vi "data_read.vi"(9 "路径":path, 10 "感情数目":dbl, 11 "训练次数":dbl) -> (0 "字符串 2":string, 2 "输出簇":T2, 3 "字符串":string)   [LabVIEW 2014]
panel:
  out "错误输出 6":errorcluster caption="错误输出"
  out "错误输出 5":errorcluster caption="错误输出"
  out "字符串 6":string
  out "字符串 5":string
  out "输出簇 4":T1
  out "错误输出 4":errorcluster caption="错误输出"
  out "错误输出 3":errorcluster caption="错误输出"
  out "字符串 4":string
  out "字符串 3":string
  out "错误输出":errorcluster
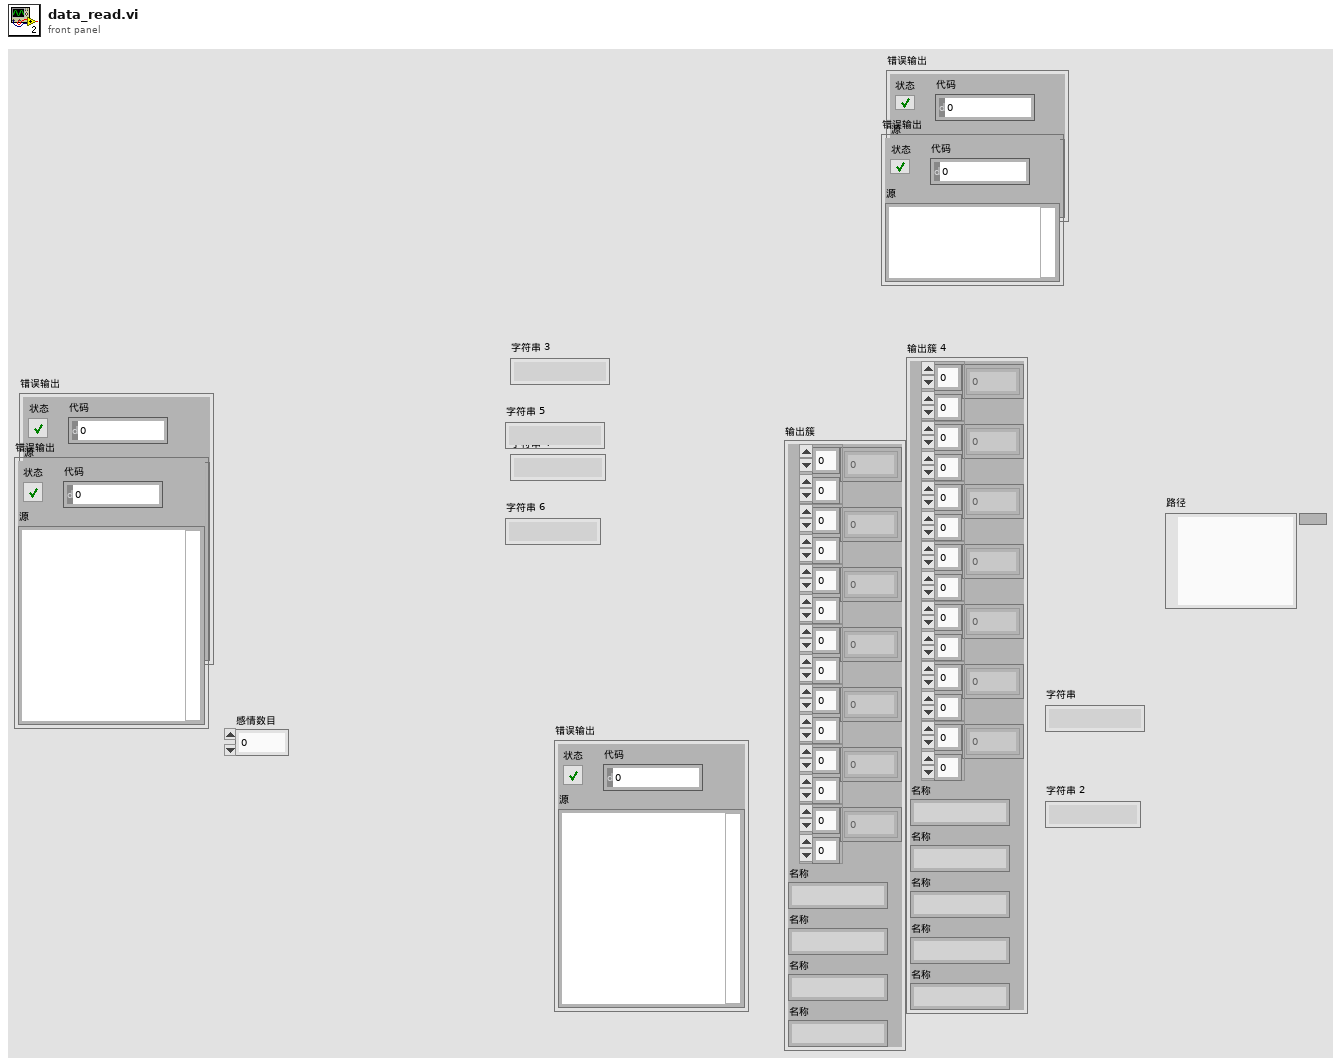
[diagram p1: front panel]
types:
  T1 = cluster{dbl[][], dbl[][], dbl[][], dbl[][], dbl[][], dbl[][], dbl[][], "名称":string, "名称":string, "名称":string, "名称":string, "名称":string}
  T2 = cluster{dbl[][], dbl[][], dbl[][], dbl[][], dbl[][], dbl[][], dbl[][], "名称":string, "名称":string, "名称":string, "名称":string}
  T3 = enum16{"open", "replace", "create", "open or create", "replace or create", "replace or create with confirmation"}
  T4 = cluster{dbl[][], dbl[][], dbl[][], dbl[][], dbl[][], dbl[][], dbl[][], "名称":string, "名称":string, "名称":string, "名称":string, "名称":string, "名称":string}
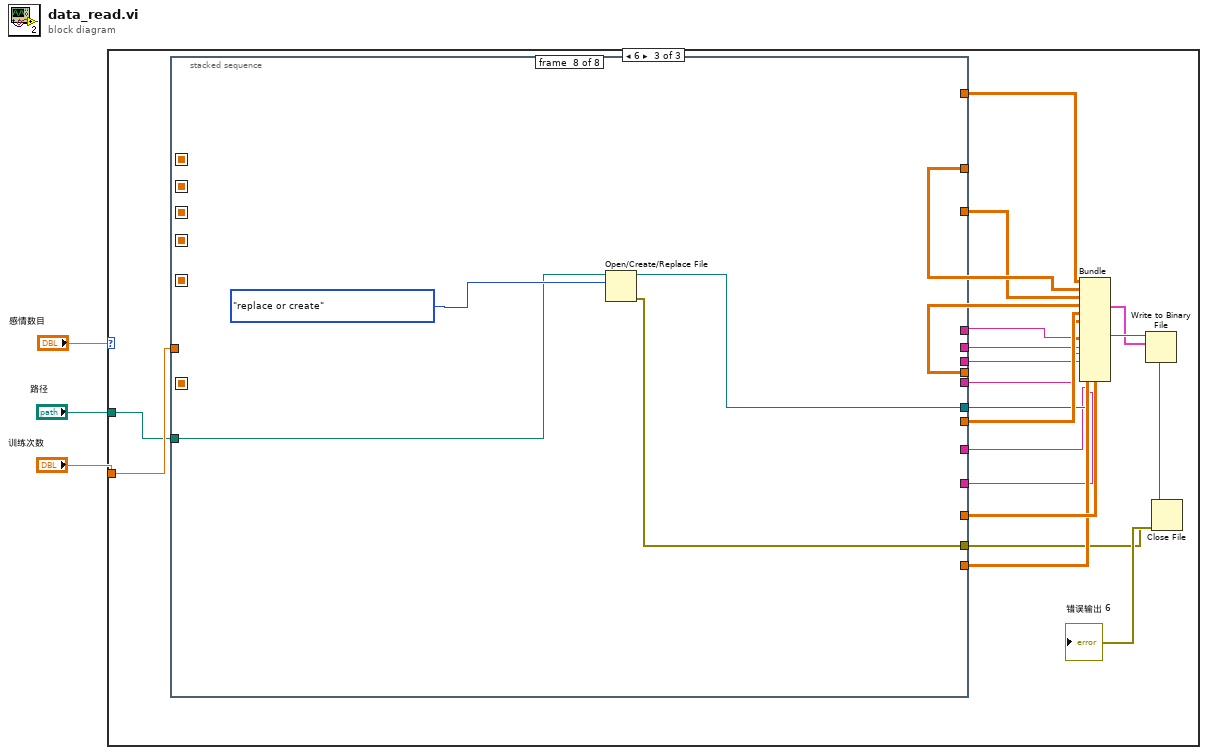
[diagram p0: block diagram]
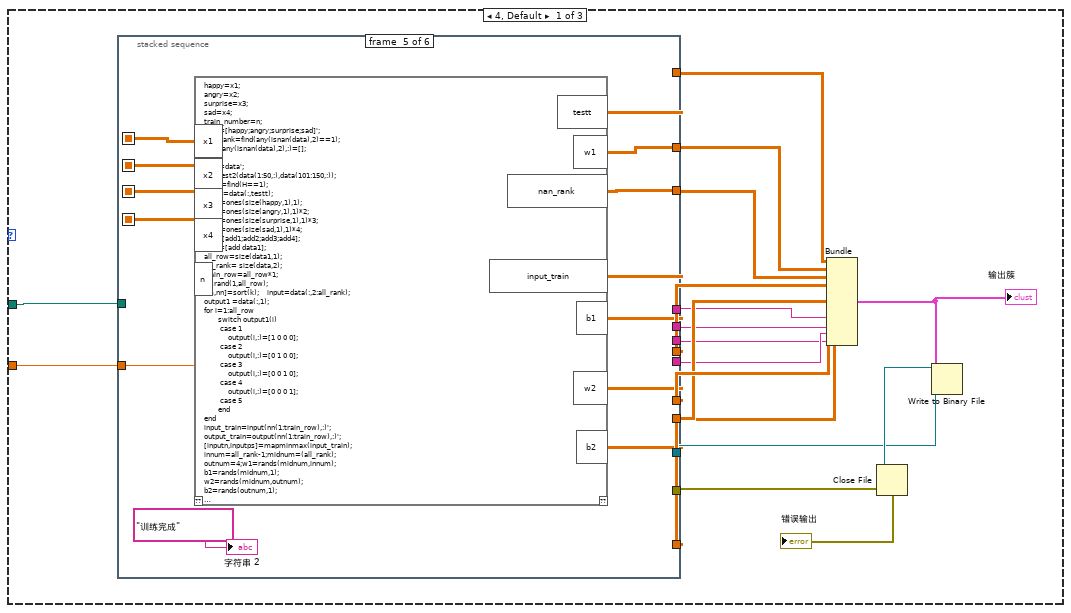
[diagram p2: hidden frame]
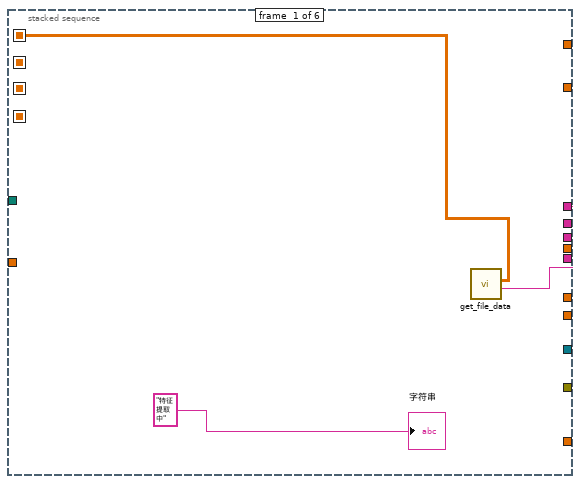
[diagram p3: hidden frame]
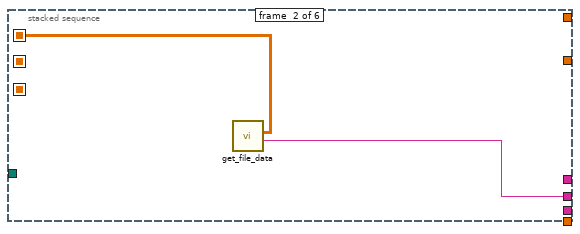
[diagram p4: hidden frame]
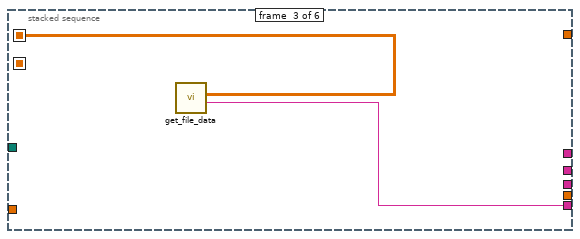
[diagram p5: hidden frame]
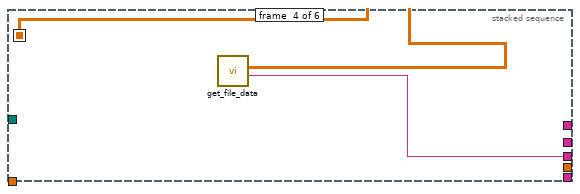
[diagram p6: hidden frame]
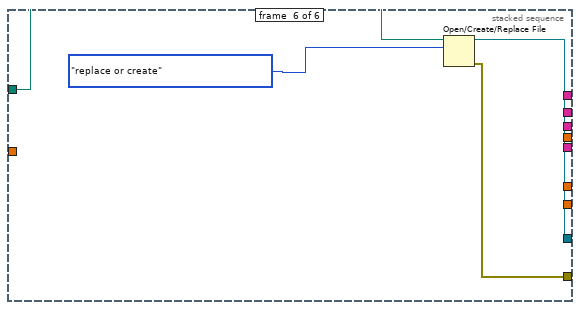
[diagram p7: hidden frame]
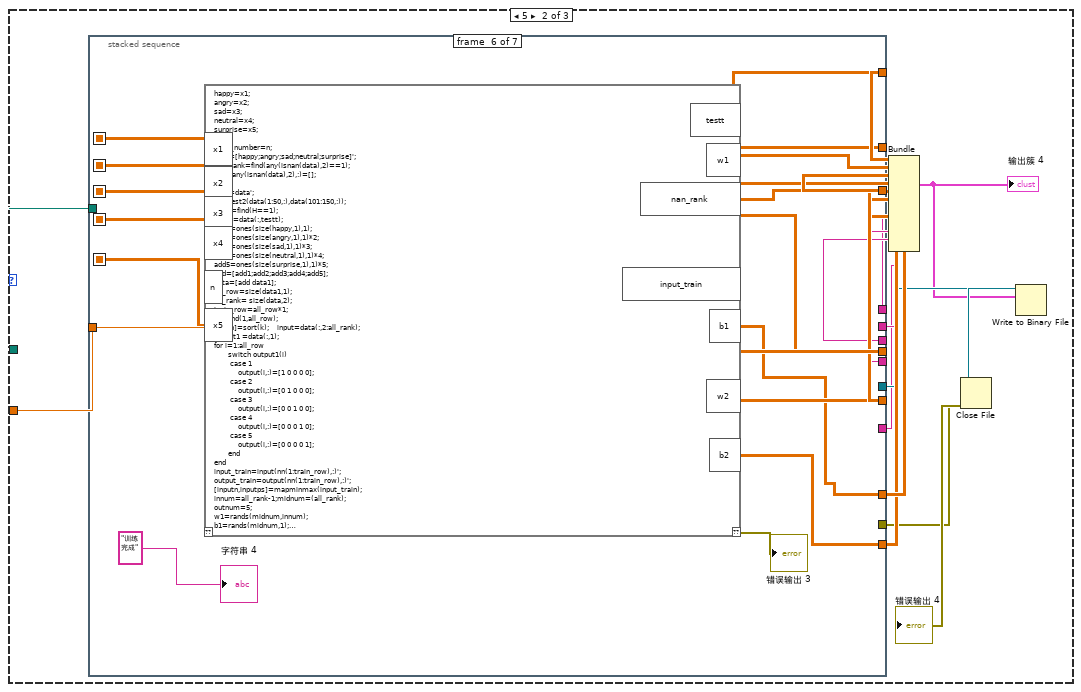
[diagram p8: hidden frame]
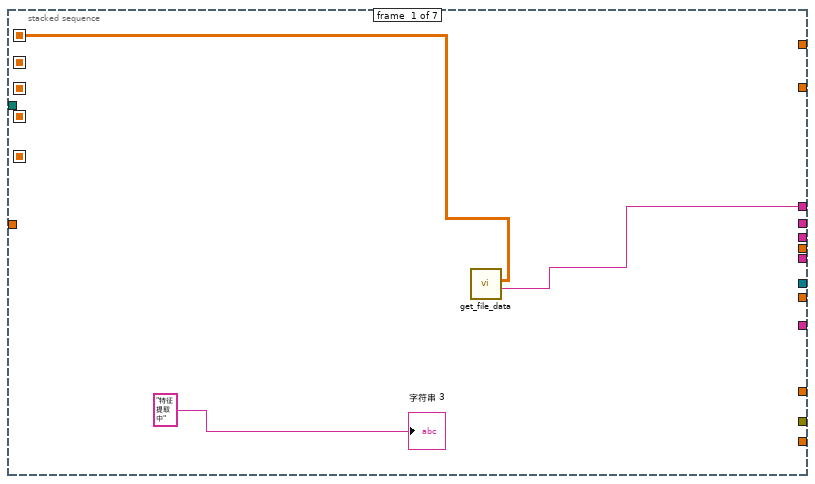
[diagram p9: hidden frame]
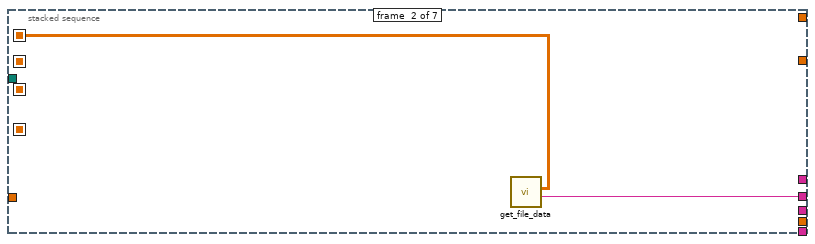
[diagram p10: hidden frame]
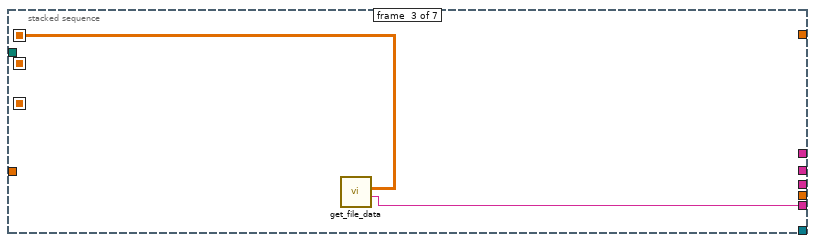
[diagram p11: hidden frame]
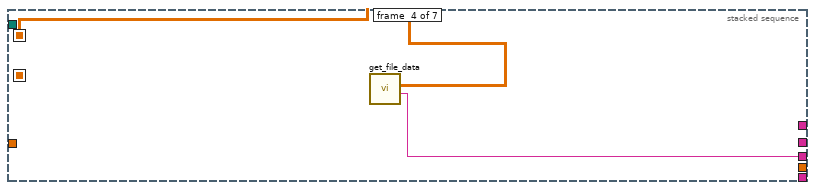
[diagram p12: hidden frame]
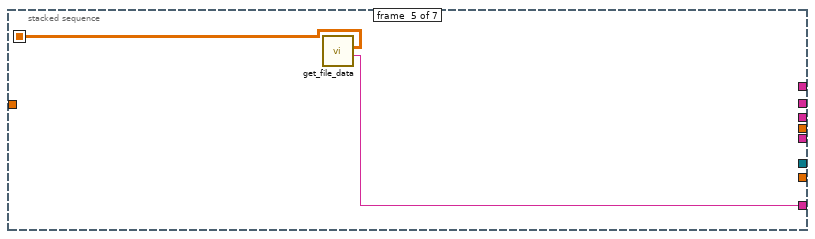
[diagram p13: hidden frame]
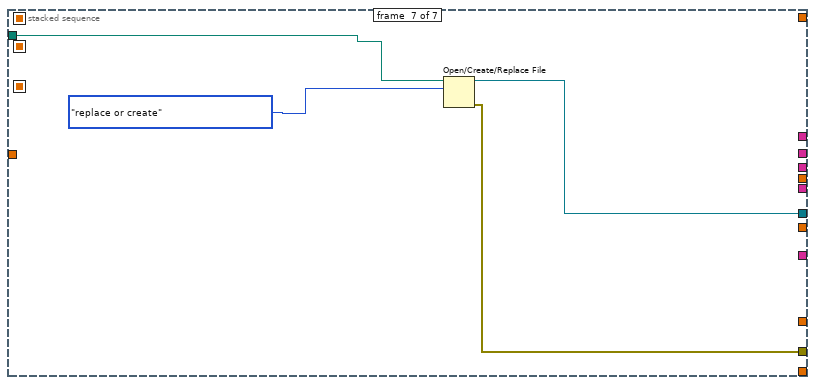
[diagram p14: hidden frame]
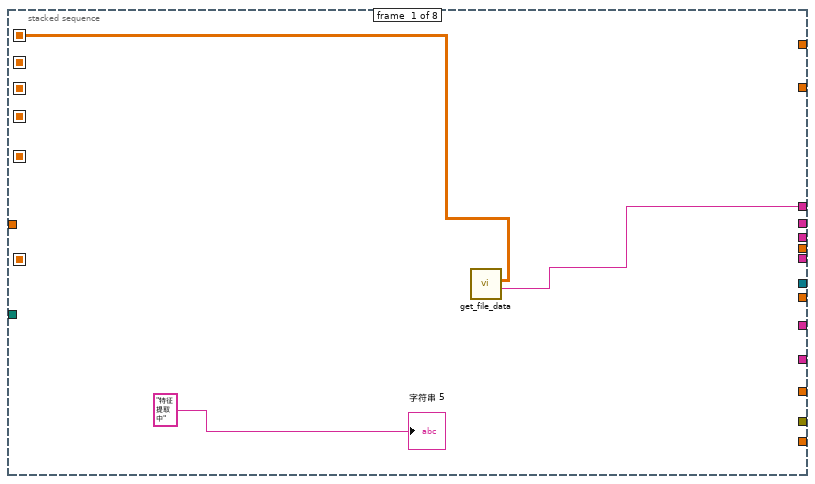
[diagram p15: hidden frame]
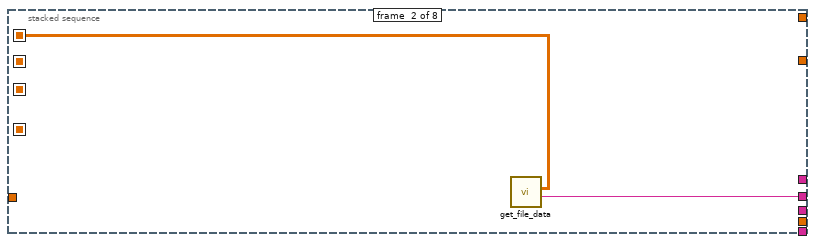
[diagram p16: hidden frame]
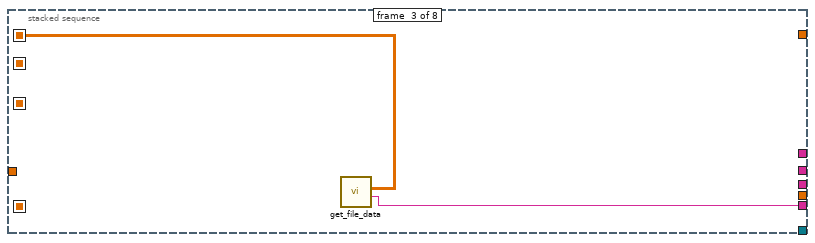
[diagram p17: hidden frame]
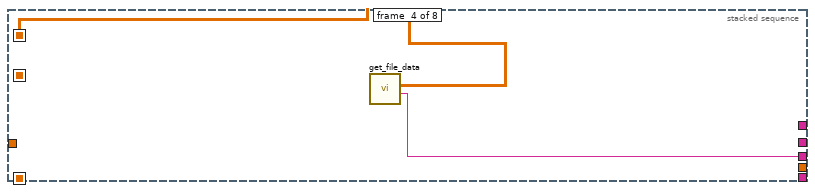
[diagram p18: hidden frame]
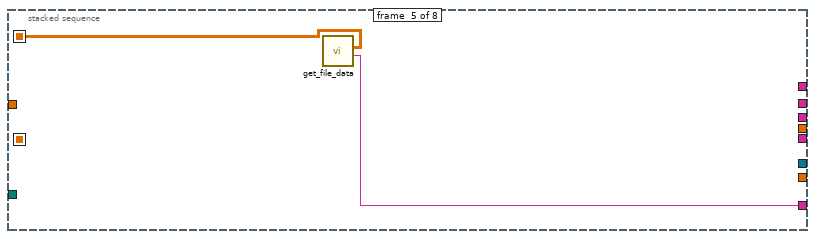
[diagram p19: hidden frame]
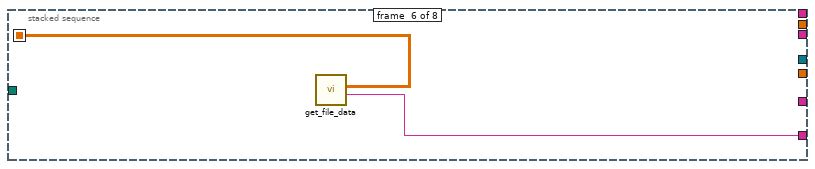
[diagram p20: hidden frame]
diagram:
  n1 = case "条件结构" shown="6" "感情数目" {
    tunnel: "训练次数" -> [w5 w50 w99]
    tunnel: "路径" -> [w4 w48 w97]
    frame 4, Default {
      n2 = stacked-sequence {
        seq-local: [w24 _ _ _ _ _] -> [_ _ _ _ w42 _]
        seq-local: [_ w26 _ _ _ _] -> [_ _ _ _ w41 _]
        seq-local: [_ _ w28 _ _ _] -> [_ _ _ _ w40 _]
        seq-local: [_ _ _ w30 _ _] -> [_ _ _ _ w43 _]
        tunnel: [_ _ _ _ w38 _] -> w20
        tunnel: w5 -> [_ _ _ _ w39 _]
        tunnel: [_ _ _ _ w32 _] -> w16
        tunnel: [_ _ _ _ w37 _] -> w18
        tunnel: [_ _ _ _ w36 _] -> w19
        tunnel: [_ _ _ _ w35 _] -> w17
        tunnel: [_ _ _ _ w34 _] -> w15
        tunnel: [_ _ _ _ w33 _] -> w21
        tunnel: [_ _ _ _ _ w46] -> w11
        tunnel: [_ _ _ _ _ w45] -> w12
        tunnel: [_ w25 _ _ _ _] -> w8
        tunnel: [_ _ w27 _ _ _] -> w9
        tunnel: [_ _ _ w29 _ _] -> w7
        tunnel: [w23 _ _ _ _ _] -> w6
        tunnel: w4 -> [_ _ _ _ _ w44]
        frame #0 {
          n3 = call "get_file_data.vi"() -> ("名称"=w23:string, "数组"=w24:dbl[][])  [unwired: 10 in]
          "字符串" <- "特征提取中"
        }
        frame #1 {
          n4 = call "get_file_data.vi"() -> ("名称"=w25:string, "数组"=w26:dbl[][])  [unwired: 10 in]
        }
        frame #2 {
          n5 = call "get_file_data.vi"() -> ("名称"=w27:string, "数组"=w28:dbl[][])  [unwired: 10 in]
        }
        frame #3 {
          n6 = call "get_file_data.vi"() -> ("名称"=w29:string, "数组"=w30:dbl[][])  [unwired: 10 in]
        }
        frame #4 {
          n7 = script code="happy=x1;\nangry=x2;\nsurprise=x3;\nsad=x4;\ntrain_number=n;\ndata=[happy;angry;surprise;sad]';\nnan_rank=find(any(isnan(data),2)==1);\ndata(any(isnan(data),2),:)=[];\n\ndata=data';\nH=ttest2(data(1:50,:),data(101:150,:));\ntestt=find(H==1);\ndata1=data(:,testt);\nadd1=ones(size(happy,1),1);\nadd2=ones(size(angry,1),1)*2;\nadd3=ones(size(surprise,1),1)*3;\nadd4=ones(size(sad,1),1)*4;\nadd=[add1;add2;add3;add4];\ndata=[add data1];\nall_row=size(data1,1);\nall_rank= size(data,2);\ntrain_row=all_row*1;\nk=rand(1,all_row);\n[m,nn]=sort(k);    input=data(:,2:all_rank);\noutput1 =data(:,1);\nfor i=1:all_row\n       switch output1(i)\n        case 1\n            output(i,:)=[1 0 0 0];\n        case 2\n            output(i,:)=[0 1 0 0];\n        case 3\n            output(i,:)=[0 0 1 0];\n        case 4\n            output(i,:)=[0 0 0 1];\n        case 5\n       end\nend\ninput_train=input(nn(1:train_row),:)';\noutput_train=output(nn(1:train_row),:)';\n[inputn,inputps]=mapminmax(input_train);\ninnum=all_rank-1;midnum=(all_rank);\noutnum=4;w1=rands(midnum,innum);\nb1=rands(midnum,1);\nw2=rands(midnum,outnum);\nb2=rands(outnum,1);\n\nw2_1=w2;w2_2=w2_1;\nw1_1=w1;w1_2=w1_1;\nb1_1=b1;b1_2=b1_1;\nb2_1=b2;b2_2=b2_1;\n\n%学习率\nxite=0.1;\nalfa=0.01;\nfor ii=1:train_number\n   \n    E(ii)=0;\n    for i=1:1:train_row\n       %% 网络预测输出 \n        x=inputn(:,i);\n        % 隐含层输出\n        for j=1:1:midnum\n            I(j)=inputn(:,i)'*w1(j,:)'+b1(j);\n            Iout(j)=1/(1+exp(-I(j)));\n        end\n        % 输出层输出\n        yn=w2'*Iout'+b2;\n        \n       %% 权值阀值修正\n        %计算误差\n        e=output_train(:,i)-yn;     \n        E(ii)=E(ii)+sum(abs(e));\n        \n        %计算权值变化率\n        dw2=e*Iout;\n        db2=e';\n        \n        for j=1:1:midnum\n            S=1/(1+exp(-I(j)));\n            FI(j)=S*(1-S);\n        end      \n        for k=1:1:innum\n            for j=1:1:midnum\n                dw1(k,j)=FI(j)*x(k)*(e(1)*w2(j,1)+e(2)*w2(j,2)+e(3)*w2(j,3)+e(4)*w2(j,4));\n                db1(j)=FI(j)*(e(1)*w2(j,1)+e(2)*w2(j,2)+e(3)*w2(j,3)+e(4)*w2(j,4));\n            end\n        end\n           \n        w1=w1_1+xite*dw1'+alfa*(w1_1-w1_2);\n        b1=b1_1+xite*db1'+alfa*(b1_1-b1_2);\n        w2=w2_1+xite*dw2'+alfa*(w2_1-w2_2);\n        b2=b2_1+xite*db2'+alfa*(b2_1-b2_2);\n        \n        w1_2=w1_1;w1_1=w1;\n        w2_2=w2_1;w2_1=w2;\n        b1_2=b1_1;b1_1=b1;\n        b2_2=b2_1;b2_1=b2;\n    end\n\nend"("x1"=w42, "x2"=w41, "x3"=w40, "x4"=w43, "n"=w39) -> ("w1"=w38:dbl[][], "b1"=w32:dbl[][], "input_train"=w37:dbl[][], "nan_rank"=w36:dbl[][], "w2"=w35:dbl[][], "b2"=w34:dbl[][], "testt"=w33:dbl[][])  [unwired: 1 in, 1 out]
          "字符串 2" <- "训练完成"
        }
        frame #5 {
          n8 = Open/Create/Replace File(file path (use dialog)=w44, operation (0:open)=T3."replace or create") -> (refnum out=w46:refnum<file>, error out=w45:errorcluster)  [unwired: 4 in, 1 out]
        }
      }
      n9 = Bundle(w21, w20, w19, w18, w17, w16, w15, "名称"=w6, "名称"=w8, "名称"=w9, "名称"=w7) -> (w10:T2)  [unwired: 1 in]
      "输出簇" <- w10
      n10 = Write to Binary File(file (use dialog)=w11, data=w10) -> (refnum out=w14:refnum<file>)  [unwired: 4 in, 2 out]
      n11 = Close File(refnum=w14, error in=w12) -> (error out=→"错误输出":errorcluster)  [unwired: 1 out]
    }
    frame 5 {
      n12 = stacked-sequence {
        seq-local: [w69 _ _ _ _ _ _] -> [_ _ _ _ _ w91 _]
        seq-local: [_ w71 _ _ _ _ _] -> [_ _ _ _ _ w90 _]
        seq-local: [_ _ w73 _ _ _ _] -> [_ _ _ _ _ w89 _]
        seq-local: [_ _ _ w75 _ _ _] -> [_ _ _ _ _ w92 _]
        seq-local: [_ _ _ _ w77 _ _] -> [_ _ _ _ _ w78 _]
        tunnel: [_ _ _ _ _ w86 _] -> w65
        tunnel: w50 -> [_ _ _ _ _ w88 _]
        tunnel: [_ _ _ _ _ w80 _] -> w61
        tunnel: [_ _ _ _ _ w85 _] -> w63
        tunnel: [_ _ _ _ _ w84 _] -> w64
        tunnel: [_ _ _ _ _ w83 _] -> w62
        tunnel: [_ _ _ _ _ w82 _] -> w60
        tunnel: [_ _ _ _ _ w81 _] -> w66
        tunnel: [_ _ _ _ _ _ w95] -> w56
        tunnel: [_ _ _ _ _ _ w94] -> w57
        tunnel: [_ w70 _ _ _ _ _] -> w53
        tunnel: [_ _ w72 _ _ _ _] -> w54
        tunnel: [_ _ _ w74 _ _ _] -> w52
        tunnel: [w68 _ _ _ _ _ _] -> w51
        tunnel: [_ _ _ _ w76 _ _] -> w49
        tunnel: w48 -> [_ _ _ _ _ _ w93]
        frame #0 {
          n13 = call "get_file_data.vi"() -> ("名称"=w68:string, "数组"=w69:dbl[][])  [unwired: 10 in]
          "字符串 3" <- "特征提取中"
        }
        frame #1 {
          n14 = call "get_file_data.vi"() -> ("名称"=w70:string, "数组"=w71:dbl[][])  [unwired: 10 in]
        }
        frame #2 {
          n15 = call "get_file_data.vi"() -> ("名称"=w72:string, "数组"=w73:dbl[][])  [unwired: 10 in]
        }
        frame #3 {
          n16 = call "get_file_data.vi"() -> ("名称"=w74:string, "数组"=w75:dbl[][])  [unwired: 10 in]
        }
        frame #4 {
          n17 = call "get_file_data.vi"() -> ("名称"=w76:string, "数组"=w77:dbl[][])  [unwired: 10 in]
        }
        frame #5 {
          n18 = script code="happy=x1;\nangry=x2;\nsad=x3;\nneutral=x4;\nsurprise=x5;\n\ntrain_number=n;\ndata=[happy;angry;sad;neutral;surprise]';\nnan_rank=find(any(isnan(data),2)==1);\ndata(any(isnan(data),2),:)=[];\n\ndata=data';\nH=ttest2(data(1:50,:),data(101:150,:));\ntestt=find(H==1);\ndata1=data(:,testt);\nadd1=ones(size(happy,1),1);\nadd2=ones(size(angry,1),1)*2;\nadd3=ones(size(sad,1),1)*3;\nadd4=ones(size(neutral,1),1)*4;\nadd5=ones(size(surprise,1),1)*5;\nadd=[add1;add2;add3;add4;add5];\ndata=[add data1];\nall_row=size(data1,1);\nall_rank= size(data,2);\ntrain_row=all_row*1;\nk=rand(1,all_row);\n[m,nn]=sort(k);    input=data(:,2:all_rank);\noutput1 =data(:,1);\nfor i=1:all_row\n       switch output1(i)\n        case 1\n            output(i,:)=[1 0 0 0 0];\n        case 2\n            output(i,:)=[0 1 0 0 0];\n        case 3\n            output(i,:)=[0 0 1 0 0];\n        case 4\n            output(i,:)=[0 0 0 1 0];\n        case 5\n            output(i,:)=[0 0 0 0 1];\n       end\nend\ninput_train=input(nn(1:train_row),:)';\noutput_train=output(nn(1:train_row),:)';\n[inputn,inputps]=mapminmax(input_train);\ninnum=all_rank-1;midnum=(all_rank);\noutnum=5;\nw1=rands(midnum,innum);\nb1=rands(midnum,1);\nw2=rands(midnum,outnum);\nb2=rands(outnum,1);\n\nw2_1=w2;w2_2=w2_1;\nw1_1=w1;w1_2=w1_1;\nb1_1=b1;b1_2=b1_1;\nb2_1=b2;b2_2=b2_1;\n\n%学习率\nxite=0.1;\nalfa=0.01;\nfor ii=1:train_number\n   \n    E(ii)=0;\n    for i=1:1:train_row\n       %% 网络预测输出 \n        x=inputn(:,i);\n        % 隐含层输出\n        for j=1:1:midnum\n            I(j)=inputn(:,i)'*w1(j,:)'+b1(j);\n            Iout(j)=1/(1+exp(-I(j)));\n        end\n        % 输出层输出\n        yn=w2'*Iout'+b2;\n        \n       %% 权值阀值修正\n        %计算误差\n        e=output_train(:,i)-yn;     \n        E(ii)=E(ii)+sum(abs(e));\n        \n        %计算权值变化率\n        dw2=e*Iout;\n        db2=e';\n        \n        for j=1:1:midnum\n            S=1/(1+exp(-I(j)));\n            FI(j)=S*(1-S);\n        end      \n        for k=1:1:innum\n            for j=1:1:midnum\n                dw1(k,j)=FI(j)*x(k)*(e(1)*w2(j,1)+e(2)*w2(j,2)+e(3)*w2(j,3)+e(4)*w2(j,4));\n                db1(j)=FI(j)*(e(1)*w2(j,1)+e(2)*w2(j,2)+e(3)*w2(j,3)+e(4)*w2(j,4));\n            end\n        end\n           \n        w1=w1_1+xite*dw1'+alfa*(w1_1-w1_2);\n        b1=b1_1+xite*db1'+alfa*(b1_1-b1_2);\n        w2=w2_1+xite*dw2'+alfa*(w2_1-w2_2);\n        b2=b2_1+xite*db2'+alfa*(b2_1-b2_2);\n        \n        w1_2=w1_1;w1_1=w1;\n        w2_2=w2_1;w2_1=w2;\n        b1_2=b1_1;b1_1=b1;\n        b2_2=b2_1;b2_1=b2;\n    end\n\nend"("x1"=w91, "x2"=w90, "x3"=w89, "x4"=w92, "n"=w88, "x5"=w78) -> ("??"=→"错误输出 3":errorcluster, "w1"=w86:dbl[][], "b1"=w80:dbl[][], "input_train"=w85:dbl[][], "nan_rank"=w84:dbl[][], "w2"=w83:dbl[][], "b2"=w82:dbl[][], "testt"=w81:dbl[][])  [unwired: 1 in]
          "字符串 4" <- "训练完成"
        }
        frame #6 {
          n19 = Open/Create/Replace File(file path (use dialog)=w93, operation (0:open)=T3."replace or create") -> (refnum out=w95:refnum<file>, error out=w94:errorcluster)  [unwired: 4 in, 1 out]
        }
      }
      n20 = Bundle(w66, w65, w64, w63, w62, w61, w60, "名称"=w51, "名称"=w53, "名称"=w54, "名称"=w52, "名称"=w49) -> (w55:T1)  [unwired: 1 in]
      "输出簇 4" <- w55
      n21 = Write to Binary File(file (use dialog)=w56, data=w55) -> (refnum out=w59:refnum<file>)  [unwired: 4 in, 2 out]
      n22 = Close File(refnum=w59, error in=w57) -> (error out=→"错误输出 4":errorcluster)  [unwired: 1 out]
    }
    frame 6 {
      n23 = stacked-sequence {
        seq-local: [w119 _ _ _ _ _ _ _] -> [_ _ _ _ _ _ w144 _]
        seq-local: [_ w121 _ _ _ _ _ _] -> [_ _ _ _ _ _ w143 _]
        seq-local: [_ _ w123 _ _ _ _ _] -> [_ _ _ _ _ _ w142 _]
        seq-local: [_ _ _ w125 _ _ _ _] -> [_ _ _ _ _ _ w145 _]
        seq-local: [_ _ _ _ w127 _ _ _] -> [_ _ _ _ _ _ w131 _]
        seq-local: [_ _ _ _ _ w128 _ _] -> [_ _ _ _ _ _ w130 _]
        tunnel: [_ _ _ _ _ _ w139 _] -> w115
        tunnel: w99 -> [_ _ _ _ _ _ w141 _]
        tunnel: [_ _ _ _ _ _ w133 _] -> w111
        tunnel: [_ _ _ _ _ _ w138 _] -> w113
        tunnel: [_ _ _ _ _ _ w137 _] -> w114
        tunnel: [_ _ _ _ _ _ w136 _] -> w112
        tunnel: [_ _ _ _ _ _ w135 _] -> w110
        tunnel: [_ _ _ _ _ _ w134 _] -> w116
        tunnel: [_ _ _ _ _ _ _ w148] -> w106
        tunnel: [_ _ _ _ _ _ _ w147] -> w107
        tunnel: [_ w120 _ _ _ _ _ _] -> w103
        tunnel: [_ _ w122 _ _ _ _ _] -> w104
        tunnel: [_ _ _ w124 _ _ _ _] -> w102
        tunnel: [w118 _ _ _ _ _ _ _] -> w101
        tunnel: [_ _ _ _ w126 _ _ _] -> w100
        tunnel: [_ _ _ _ _ w129 _ _] -> w98
        tunnel: w97 -> [_ _ _ _ _ _ _ w146]
        frame #0 {
          n24 = call "get_file_data.vi"() -> ("名称"=w118:string, "数组"=w119:dbl[][])  [unwired: 10 in]
          "字符串 5" <- "特征提取中"
        }
        frame #1 {
          n25 = call "get_file_data.vi"() -> ("名称"=w120:string, "数组"=w121:dbl[][])  [unwired: 10 in]
        }
        frame #2 {
          n26 = call "get_file_data.vi"() -> ("名称"=w122:string, "数组"=w123:dbl[][])  [unwired: 10 in]
        }
        frame #3 {
          n27 = call "get_file_data.vi"() -> ("名称"=w124:string, "数组"=w125:dbl[][])  [unwired: 10 in]
        }
        frame #4 {
          n28 = call "get_file_data.vi"() -> ("名称"=w126:string, "数组"=w127:dbl[][])  [unwired: 10 in]
        }
        frame #5 {
          n29 = call "get_file_data.vi"() -> ("名称"=w129:string, "数组"=w128:dbl[][])  [unwired: 10 in]
        }
        frame #6 {
          n30 = script code="happy=x1;\nangry=x2;\nsad=x3;\nneutral=x4;\nsurprise=x5;\nfear=x6;\n\ntrain_number=n;\ndata=[happy;angry;sad;neutral;surprise;fear]';\nnan_rank=find(any(isnan(data),2)==1);\ndata(any(isnan(data),2),:)=[];\n\ndata=data';\nH=ttest2(data(1:50,:),data(101:150,:));\ntestt=find(H==1);\ndata1=data(:,testt);\nadd1=ones(size(happy,1),1);\nadd2=ones(size(angry,1),1)*2;\nadd3=ones(size(sad,1),1)*3;\nadd4=ones(size(neutral,1),1)*4;\nadd5=ones(size(surprise,1),1)*5;\nadd6=ones(size(fear,1),1)*6;\nadd=[add1;add2;add3;add4;add5;add6];\ndata=[add data1];\nall_row=size(data1,1);\nall_rank= size(data,2);\ntrain_row=all_row*1;\nk=rand(1,all_row);\n[m,nn]=sort(k);    input=data(:,2:all_rank);\noutput1 =data(:,1);\nfor i=1:all_row\n       switch output1(i)\n        case 1\n            output(i,:)=[1 0 0 0 0 0];\n        case 2\n            output(i,:)=[0 1 0 0 0 0];\n        case 3\n            output(i,:)=[0 0 1 0 0 0];\n        case 4\n            output(i,:)=[0 0 0 1 0 0];\n        case 5\n            output(i,:)=[0 0 0 0 1 0];\n        case 6\n            output(i,:)=[0 0 0 0 0 1];\n       end\nend\ninput_train=input(nn(1:train_row),:)';\noutput_train=output(nn(1:train_row),:)';\n[inputn,inputps]=mapminmax(input_train);\ninnum=all_rank-1;midnum=(all_rank);\noutnum=6;\nw1=rands(midnum,innum);\nb1=rands(midnum,1);\nw2=rands(midnum,outnum);\nb2=rands(outnum,1);\n\nw2_1=w2;w2_2=w2_1;\nw1_1=w1;w1_2=w1_1;\nb1_1=b1;b1_2=b1_1;\nb2_1=b2;b2_2=b2_1;\n\n%学习率\nxite=0.1;\nalfa=0.01;\nfor ii=1:train_number\n   \n    E(ii)=0;\n    for i=1:1:train_row\n       %% 网络预测输出 \n        x=inputn(:,i);\n        % 隐含层输出\n        for j=1:1:midnum\n            I(j)=inputn(:,i)'*w1(j,:)'+b1(j);\n            Iout(j)=1/(1+exp(-I(j)));\n        end\n        % 输出层输出\n        yn=w2'*Iout'+b2;\n        \n       %% 权值阀值修正\n        %计算误差\n        e=output_train(:,i)-yn;     \n        E(ii)=E(ii)+sum(abs(e));\n        \n        %计算权值变化率\n        dw2=e*Iout;\n        db2=e';\n        \n        for j=1:1:midnum\n            S=1/(1+exp(-I(j)));\n            FI(j)=S*(1-S);\n        end      \n        for k=1:1:innum\n            for j=1:1:midnum\n                dw1(k,j)=FI(j)*x(k)*(e(1)*w2(j,1)+e(2)*w2(j,2)+e(3)*w2(j,3)+e(4)*w2(j,4));\n                db1(j)=FI(j)*(e(1)*w2(j,1)+e(2)*w2(j,2)+e(3)*w2(j,3)+e(4)*w2(j,4));\n            end\n        end\n           \n        w1=w1_1+xite*dw1'+alfa*(w1_1-w1_2);\n        b1=b1_1+xite*db1'+alfa*(b1_1-b1_2);\n        w2=w2_1+xite*dw2'+alfa*(w2_1-w2_2);\n        b2=b2_1+xite*db2'+alfa*(b2_1-b2_2);\n        \n        w1_2=w1_1;w1_1=w1;\n        w2_2=w2_1;w2_1=w2;\n        b1_2=b1_1;b1_1=b1;\n        b2_2=b2_1;b2_1=b2;\n    end\n\nend"("x1"=w144, "x2"=w143, "x3"=w142, "x4"=w145, "n"=w141, "x5"=w131, "x6"=w130) -> ("??"=→"错误输出 5":errorcluster, "w1"=w139:dbl[][], "b1"=w133:dbl[][], "input_train"=w138:dbl[][], "nan_rank"=w137:dbl[][], "w2"=w136:dbl[][], "b2"=w135:dbl[][], "testt"=w134:dbl[][])  [unwired: 1 in]
          "字符串 6" <- "训练完成"
        }
        frame #7 {
          n31 = Open/Create/Replace File(file path (use dialog)=w146, operation (0:open)=T3."replace or create") -> (refnum out=w148:refnum<file>, error out=w147:errorcluster)  [unwired: 4 in, 1 out]
        }
      }
      n32 = Bundle(w116, w115, w114, w113, w112, w111, w110, "名称"=w101, "名称"=w103, "名称"=w104, "名称"=w102, "名称"=w100, "名称"=w98) -> (w105:T4)  [unwired: 1 in]
      n33 = Write to Binary File(file (use dialog)=w106, data=w105) -> (refnum out=w109:refnum<file>)  [unwired: 4 in, 2 out]
      n34 = Close File(refnum=w109, error in=w107) -> (error out=→"错误输出 6":errorcluster)  [unwired: 1 out]
    }
  }
